vi "Read controller_.vi"(8 "error in (no error)":errorcluster, 11 "Configurable Device in":refnum<class "Configurable Device.lvclass">) -> (0 "error out":errorcluster, 2 "controller?":bool, 3 "Configurable Device out":refnum<class "Configurable Device.lvclass">)   [LabVIEW 2016, in "Configurable Device.lvclass"]
uses:
  Configurable Device.lvclass
  Configurable Device.lvclass/Configurable Device.ctl
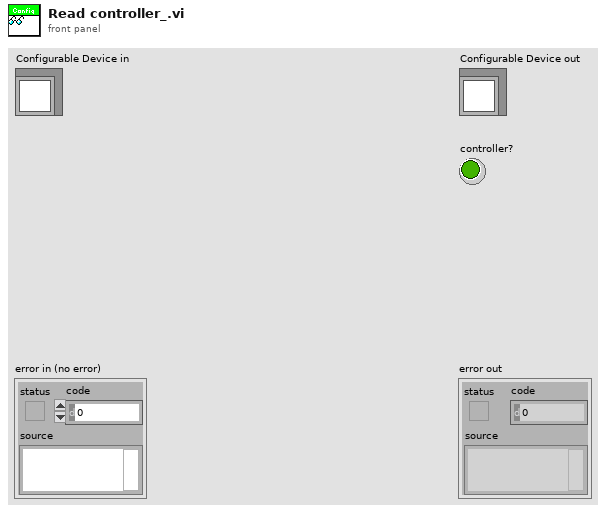
[diagram p1: front panel]
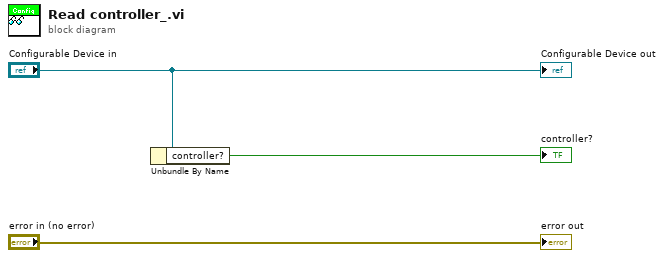
[diagram p0: block diagram]
diagram:
  n1 = Unbundle By Name("Configurable Device in") -> ("controller?"=→"controller?":bool)
  "error out" <- "error in (no error)"
  "Configurable Device out" <- "Configurable Device in"
